vi "AlliGator Toggle Phasor Plot(s) Locking to Reference n.vi"(4 "Ref 1(F)/Ref 2(T)":bool, 6 "Phasor Frequency":dbl[unit], 7 "Phasor Graph Refnum":refnum<vi>, 8 "error in":errorcluster, 9 "State Indicators":refnum<vi>, 10 "Phasor Graph Ctrl Refnums":T1, 11 "[Phasor Plot(s) locked to Ref n] in":i32[](array[numeric])) -> (0 "error out":errorcluster, 3 "[Phasor Plot(s) locked to Ref n] out":i32[](array[numeric]))   [LabVIEW 2021, in "AlliGator Phasor Graph.lvlib"]
doc: "Locks Phasor Plot(s) to a reference."
uses:
  AlliGator Phasor Graph.lvlib
  GUI/AlliGator Phasor Graph Ctrl Refnums.ctl
  Phasor/Phasor Calibration Type.ctl
  GUI/AlliGator State Indicator.ctl
  Globals, Variables, Constants/AlliGator Variables List.ctl
  Globals, Variables, Constants/AlliGator Globals, Variables & Constants.lvlib
  Graphs/XY Graph/XY Graph Add-Ons.lvlib
  Sound/Sound.lvlib
  Phasor/Phasor.lvlib
  GUI/AlliGator GUI.lvlib
panel:
  # "see the AlliGator License on the block diagram (Ctrl+E or Window:Show Block Diagram)"
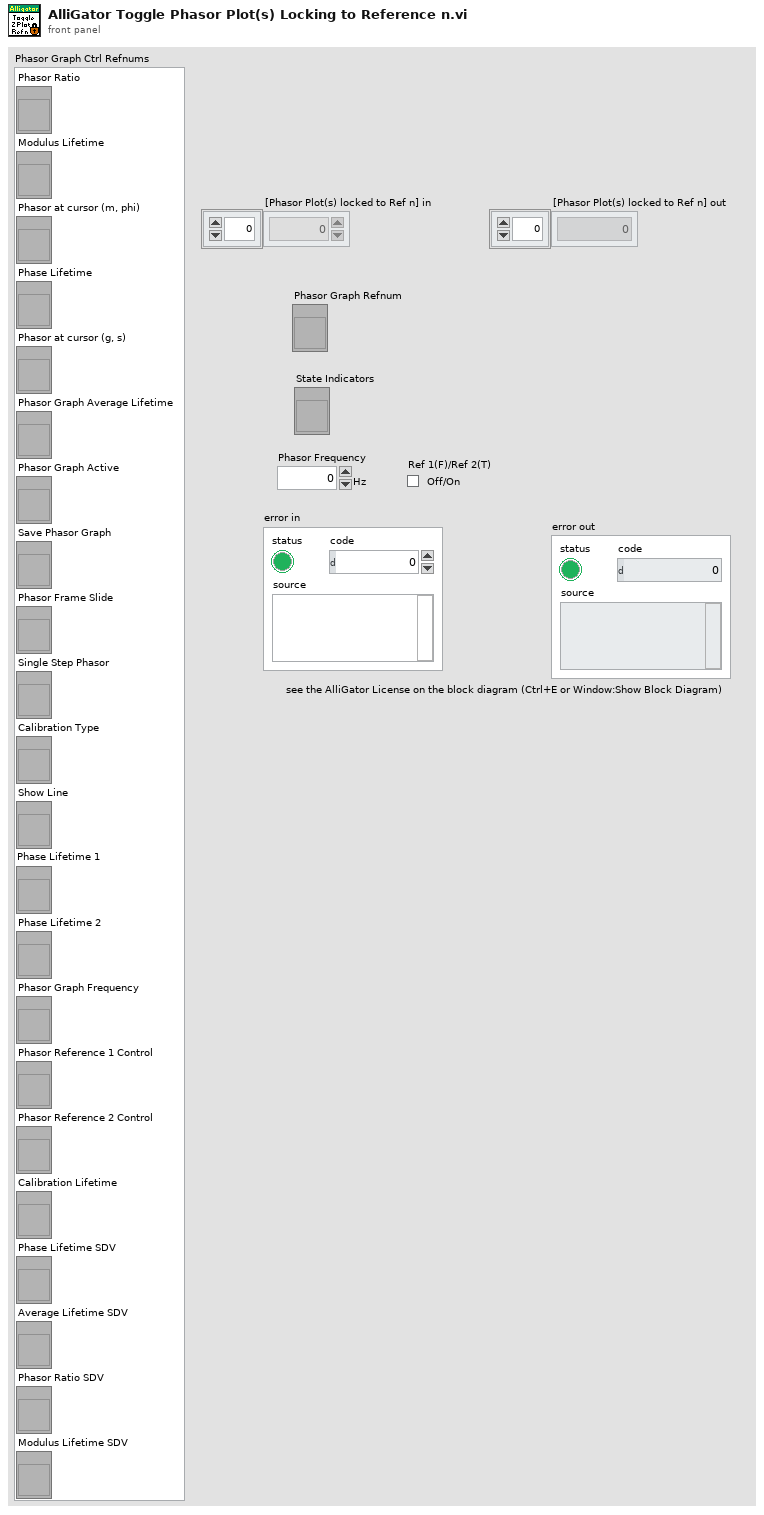
[diagram p1: front panel]
types:
  T1 = typedef "AlliGator GUI.lvlib/AlliGator Phasor Graph Ctrl Refnums.ctl" = cluster{"Phasor Ratio":refnum<vi>, "Modulus Lifetime":refnum<vi>, "Phasor at cursor (m, phi)":refnum<vi>, "Phase Lifetime":refnum<vi>, "Phasor at cursor (g, s)":refnum<vi>, "Phasor Graph Average Lifetime":refnum<vi>, "Phasor Graph Active":refnum<vi>, "Save Phasor Graph":refnum<vi>, "Phasor Frame Slide":refnum<vi>, "Single Step Phasor":refnum<vi>, "Calibration Type":refnum<vi>, "Show Line":refnum<vi>, "Phase Lifetime 1":refnum<vi>, "Phase Lifetime 2":refnum<vi>, "Phasor Graph Frequency":refnum<vi>, "Phasor Reference 1 Control":refnum<vi>, "Phasor Reference 2 Control":refnum<vi>, "Calibration Lifetime":refnum<vi>, "Phase Lifetime SDV":refnum<vi>, "Average Lifetime SDV":refnum<vi>, "Phasor Ratio SDV":refnum<vi>, "Modulus Lifetime SDV":refnum<vi>}
  T2 = typedef "AlliGator Globals, Variables & Constants.lvlib/AlliGator Variables List.ctl" = enum16{"---- GUI ----", "GUI:Initialization Status", "GUI:State Indicators Refnum", "GUI:Original AlliGator Menu Items", "GUI:Current Action Loop State", "GUI:Script in progress", "GUI:Playback", "GUI:Loop Playback", "GUI:Search ROI Used", "GUI:Search ROI", "Decay Graph Max Legend Size", "Intensity Graph Max Legend Size", "Decay Statistics Graph Max Legend Size", "Phasor Graph Max Legend Size", "Phasor Ratio Graph Max Legend Size", "Lifetime Graph Max Legend Size", "---- Files ----", "Files:Export Dataset Frames as Individual Files", "Files:Show Batch Export Help Balloons", "Files:Frames in Dataset", "Files:ptu File Frame Start Indices", "Files:Current Frame in Dataset", "Files:Current Frame Timestamp", "Files:Dataset Loaded", "Files:Dataset Metadata", "Files:Dataset Channel", "Files:Dataset Data Description", "Files:Background Dataset Metadata", "Files:Background Dataset Channel", "Files:Background Dataset Data Description", "Files:Background File Subtraction", "Files:Background File Path", "Files:Background File Pile-up Correction", "Files:Background File Pixel Well Capacity", "Files:Background File Scaling Factor", "Files:Current Dataset Load Settings", "Files:Dataset Path", "Files:ICCD-specific Information", "Files:Macrotime Gate Separation", "------ Python Plugins ------", "Python Plugins:Information", "Python Plugins:Python Session", "Python Plugins:Valid Python Session?", "---- Source Image ----", "Source Image:ROIs", "Source Image:Current ROI", "Source Image:ROI Event Refnum", "X_Source Image Display Range", "X_Source Image Palette Information", "X_Type of Displayed Image", "X_Time Gate Slider", "Source Image:Palette List", "Source Image:Scale", "Source Image:ROI Overlay Color", "Source Image:Overlay to Erase", "Source Image:Is Displayed Image Accumulated", "Source Image:White Light Image Modified", "Source Image:Mask Image Modified", "---- Image Profile Window ----", "Image Profile:Window Event Refnum", "Image Profile:IntensityType", "Image Profile:Intensity Average Type", "Image Profile:Intensity-weighted SDV", "Image Profile:Box Profile Type", "Image Profile:Window Open", "Image Profile:Plotted Fit Parameter", "------ Phasor Graph -------", "Phasor Graph:Show Line", "---- Phasor Plot ---", "Phasor Plot:Parameters Changed", "Phasor Plot:FLI Dataset Modified since last Calculation", "Phasor Harmonics Data", "Selected Phasor Harmonics", "Phasor Harmonic Manager Event Refnum", "Phasor Plot:ROIs", "Phasor Plot:Current ROI", "Phasor Plot:ROI Event Refnum", "Phasor Plot:Image Reference Points", "Phasor Plot:Computed", "Phasor Plot:Palette Information", "Phasor Plot:Palette List", "Phasor Plot:Phasor Ratio Palette Information", "Phasor Plot:Phasor Ratio Palette List", "Phasor Plot:Image Scale", "Phasor Plot:Image Overlay to Erase", "Phasor Plot:Image Elements to Update", "Phasor Plot:Current Calculation Parameters", "Phasor Plot:Current Calibration Options", "Phasor Plot:Reset Cumulated Phasor Plot", "Phasor Plot:Reference 1", "Phasor Plot:Lifetime Reference 1", "Phasor Plot:Reference 1 Frequency", "Phasor Plot:Reference 2", "Phasor Plot:Lifetime Reference 2", "Phasor Plot:Reference 2 Frequency", "---- Decay Analysis ----", "Number of Selected Decays to Fit", "LS Fit Results", "LAR Fit Results", "BS Fit Results", "Last Decay Max - Min", "Best Fit Parameters", "Best Fit Parameter Names", "Actual Size X", "Actual Size Y", "Binning X", "Binning Y", "Actual # Gates", "Dataset Number", "Gates to...", "Gates Skipped", "Gates to keep", "Gate Step", "Gate Separation", "Reversed Gates", "Pile-up Correction", "Pixel Well Capacity", "Background Subtracted", "Background Subtraction Method", "Background Definition Range", "Background File (deprecated)", "Number of Dataset Accumulated", "Array of Accumulated Dataset Paths", "Do Averaged Datasets", "Destination File Path", "Process Plot Target", "Use 1/D as Phasor Frequency", "---- Decay Fit Parameter Map -----", "Decay Fit Parameter Map:Palette Information", "Decay Fit Parameter Map:Palette List", "---- Parameter Map ----", "Parameter Map:Palette Information", "Parameter Map:Palette List", "------- Local Decay Window ---------", "Local Decay Graph Window:Event Refnum", "Local Decay Graph Window:Use normalized IRF for convolution", "----- Miscellaneous ----", "Misc:Skippable Dialog Windows Status"}
  T3 = typedef "AlliGator State Indicator.ctl" = cluster{"Phasor Calibration Defined":bool, "Phasor Calibration Series Defined":bool, "Phasor Calibration Map Defined":bool, "Phasor Ratio Reference 1 Defined":bool, "Phasor Ratio Reference 2 Defined":bool, "Phasor Ratio Lifetime Reference 1 Defined ":bool, "Phasor Ratio Lifetime Reference 2 Defined":bool, "Phasor Calibration Used":bool, "Phasor Calibration Series Used":bool, "Phasor Calibration Map Used":bool, "Dataset Update Needed":bool, "Phasor Plot Update Needed":bool, "Reference/IRF Defined":bool, "Individual IRFs Defined":bool}
  T4 = typedef "Phasor.lvlib/Phasor (m, phi).ctl" = cluster{"m":dbl, "phi":dbl}
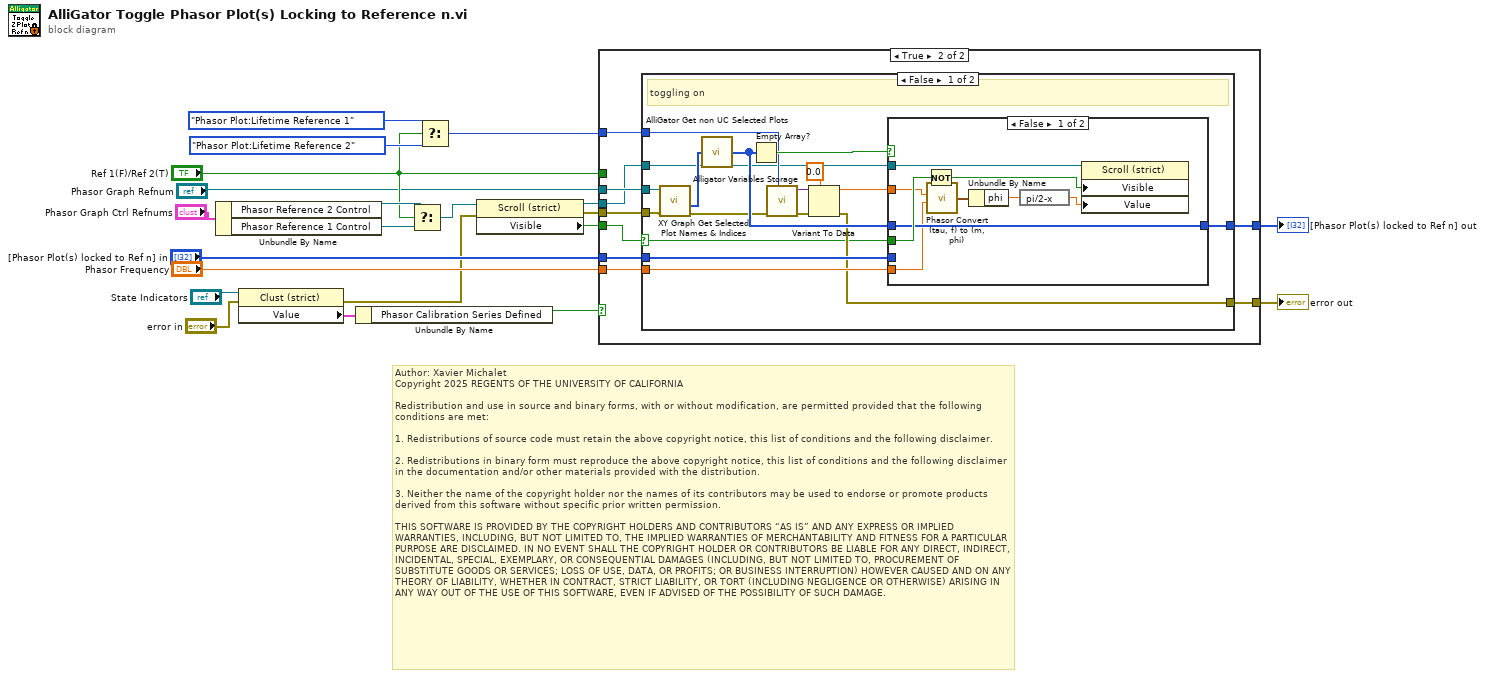
[diagram p0: block diagram]
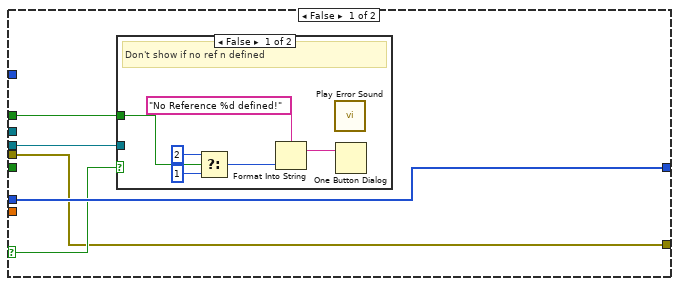
[diagram p2: hidden frame]
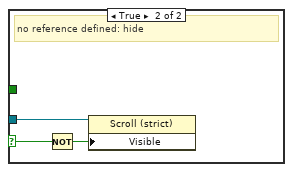
[diagram p3: hidden frame]
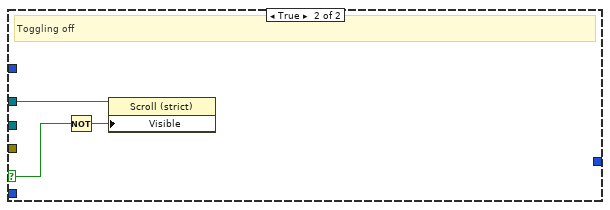
[diagram p5: hidden frame]
diagram:
  # "Author: Xavier Michalet\nCopyright 2025 REGENTS OF THE UNIVERSITY OF CALIFORNIA\n\nRedistribution and use in source and binary forms, with or without modification, are permitted provided that the following conditions are met:\n\n1. Redistributions of source code must retain the above copyright notice, this list of conditions and the following disclaimer.\n\n2. Redistributions in binary form must reproduce the above copyright notice, this list of conditions and the following disclaimer in the documentation and/or other materials provided with the distribution.\n\n3. Neither the name of the copyright holder nor the names of its contributors may be used to endorse or promote products derived from this software without specific prior written permission.\n\nTHIS SOFTWARE IS PROVIDED BY THE COPYRIGHT HOLDERS AND CONTRIBUTORS “AS IS” AND ANY EXPRESS OR IMPLIED WARRANTIES, INCLUDING, BUT NOT LIMITED TO, THE IMPLIED WARRANTIES OF MERCHANTABILITY AND FITNESS FOR A PARTICULAR PURPOSE ARE DISCLAIMED. IN NO EVENT SHALL THE COPYRIGHT HOLDER OR CONTRIBUTORS BE LIABLE FOR ANY DIRECT, INDIRECT, INCIDENTAL, SPECIAL, EXEMPLARY, OR CONSEQUENTIAL DAMAGES (INCLUDING, BUT NOT LIMITED TO, PROCUREMENT OF SUBSTITUTE GOODS OR SERVICES; LOSS OF USE, DATA, OR PROFITS; OR BUSINESS INTERRUPTION) HOWEVER CAUSED AND ON ANY THEORY OF LIABILITY, WHETHER IN CONTRACT, STRICT LIABILITY, OR TORT (INCLUDING NEGLIGENCE OR OTHERWISE) ARISING IN ANY WAY OUT OF THE USE OF THIS SOFTWARE, EVEN IF ADVISED OF THE POSSIBILITY OF SUCH DAMAGE."
  n1 = Unbundle By Name("Phasor Graph Ctrl Refnums") -> ("Phasor Reference 2 Control"=w7:refnum<vi>, "Phasor Reference 1 Control"=w8:refnum<vi>)
  n2 = property on="Property Node" class="Clust (strict)"(reference="State Indicators", error in="error in") -> (error out=w10:errorcluster, "Value"=w15:T3)  [unwired: 1 out]
  n3 = Unbundle By Name(w15) -> ("Phasor Calibration Series Defined"=w14:bool)
  n4 = Select(t=w7, s="Ref 1(F)/Ref 2(T)", f=w8) -> (s? t:f=w6:refnum<vi>)
  n5 = Select(t=AlliGator_Variables_List."Phasor Plot:Lifetime Reference 1" ("Alligator Variable"), s="Ref 1(F)/Ref 2(T)", f=AlliGator_Variables_List."Phasor Plot:Lifetime Reference 2" ("Alligator Variable")) -> (s? t:f=w3:T2)
  n6 = property on="Property Node" class="Scroll (strict)"(reference=w6, error in=w10) -> (reference out=w12:refnum<vi>, error out=w9:errorcluster, "Visible"=w13:bool)
  n7 = case shown="True" w14 {
    selector: w14 -> [w25 _]
    tunnel: "[Phasor Plot(s) locked to Ref n] in" -> [w26 w44]
    tunnel: [w26 w43] -> w19
    tunnel: "Phasor Frequency" -> [_ w42]
    tunnel: "Phasor Graph Refnum" -> [_ w41]
    tunnel: [w23 w40] -> w21
    tunnel: w13 -> [_ w39]
    tunnel: w12 -> [w24 w38]
    tunnel: w9 -> [w23 w37]
    tunnel: w3 -> [_ w36]
    tunnel: "Ref 1(F)/Ref 2(T)" -> [w22 _]
    frame False {
      n8 = case shown="False" w25 {
        selector: w25 -> [_ w35]
        tunnel: w24 -> [_ w33]
        tunnel: w22 -> [w30 _]
        frame False {
          # "Don't show if no ref n defined"
          n9 = Select(t=2, s=w30, f=1) -> (s? t:f=w27:i32)
          n10 = Format Into String(format string="No Reference %d defined!" ("message"), w27) -> (resulting string=w31:string)  [unwired: 2 in, 1 out]
          n11 = call "Play Error Sound.vi"() -> ()  [unwired: 27 in, 1 out]
          n12 = One Button Dialog(message=w31) -> ()  [unwired: 1 in, 1 out]
        }
        frame True {
          # "no reference defined: hide"
          n13 = Not(x=w35) -> (.not. x?=w34:bool)
          n14 = property on="Property Node" class="Scroll (strict)"(reference=w33, "Visible"=w34) -> ()  [unwired: 1 in, 2 out]
        }
      }
    }
    frame True {
      n15 = case shown="False" w39 {
        selector: w39 -> [w46 w72]
        tunnel: w44 -> [w60 _]
        tunnel: [w61 _] -> w43
        tunnel: w41 -> [w59 _]
        tunnel: w42 -> [w55 _]
        tunnel: w36 -> [w54 _]
        tunnel: [w49 _] -> w40
        tunnel: w38 -> [w47 w73]
        tunnel: w37 -> [w45 _]
        frame False {
          # "toggling on"
          n16 = call "XY Graph Get Selected Plot Names & Indices.vi"("error in (no error)"=w45, "XYGraph in"=w59) -> ("error out"=w48:errorcluster, "Selected Plots"=w58:i32[])  [unwired: 5 in, 3 out]
          n17 = call "AlliGator Get non UC Selected Plots.vi"("Selected Plots"=w58) -> ("Selected Plots - UC"=w56:i32[])  [unwired: 8 in]
          n18 = Empty Array?(array=w56) -> (empty?=w57:bool)
          n19 = call "Alligator Variables Storage.vi"("AlliGator Variable"=w54, "Error In"=w48) -> ("Error Out"=w52:errorcluster, "Data out"=w53:variant)  [unwired: 7 in, 1 out]
          n20 = Variant To Data(error in=w52, type=dbl[unit] 0.0 ("Lifetime"), Variant=w53) -> (data=w50:dbl[unit], error out=w49:errorcluster)
          n21 = case shown="False" w57 {
            tunnel: w46 -> [w69 _]
            tunnel: [w66 w71] -> w61
            tunnel: w60 -> [_ w71]
            tunnel: w56 -> [w66 _]
            tunnel: w55 -> [w65 _]
            tunnel: w50 -> [w64 _]
            tunnel: w47 -> [w62 _]
            frame False {
              n22 = Not(x=w69) -> (.not. x?=w70:bool)
              n23 = call "Phasor Convert (tau, f) to (m, phi).vi"("Lifetime"=w64, "Phasor Frequency"=w65) -> ("Phasor (m, phi)"=w68:T4)  [unwired: 5 in]
              n24 = Unbundle By Name(w68) -> ("phi"=w63:dbl)
              n25 = expression code="pi/2-x"(w63) -> (w67:dbl)
              n26 = property on="Property Node" class="Scroll (strict)"(reference=w62, "Visible"=w70, "Value"=w67) -> ()  [unwired: 1 in, 2 out]
            }
            frame True {
              # "UC: ignore"
            }
          }
        }
        frame True {
          # "Toggling off"
          n27 = Not(x=w72) -> (.not. x?=w74:bool)
          n28 = property on="Property Node" class="Scroll (strict)"(reference=w73, "Visible"=w74) -> ()  [unwired: 1 in, 2 out]
        }
      }
    }
  }
  "error out" <- w21
  "[Phasor Plot(s) locked to Ref n] out" <- w19
